vi "Close connection (SubVI).vi"(2 "error in (no error)":errorcluster, 3 "Connection in":refnum<class "Connection.lvclass">) -> (0 "error out":errorcluster)   [LabVIEW 2016]
uses:
  <vilib>/Distrio/LabbitMQ/Connection/Connection.lvclass
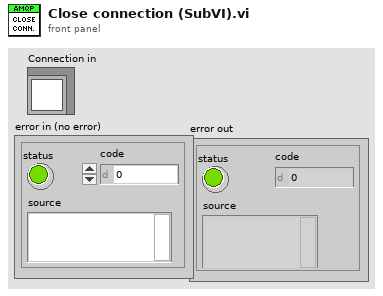
[diagram p1: front panel]
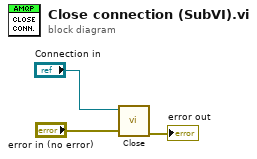
[diagram p0: block diagram]
diagram:
  n1 = call <vilib>:"Close.vi"("error in (no error)"="error in (no error)", "Connection in"="Connection in") -> ("error out"=→"error out":errorcluster)  [unwired: 8 in, 1 out]
